vi "PDSS - New Trigger Sequence - Calculate Complete Line Scan.vi"(8 "error in":errorcluster, 9 "FPS":dbl=30.0 format="%0.2p", 10 "Modulation Cycles\nAt Each Wavelength":dbl=1.0 min=1.0 max=30.0 step=1.0, 11 "LCVR Voltages":dbl[][](array[numeric])=[[0.0, 0.0, 0.0, 1.0]]) -> (0 "error out":errorcluster, 1 "LCVR Relaxtion Time":dbl=200.0 format="%#_13g", 3 "AO Graph":waveform(dbl)[](graph)=[{"t0"=timestamp(0 s since 1904-01-01), "dt"=0.000125, "Y"=array[2667 elements]}, {"t0"=timestamp(0 s since 1904-01-01), "dt"=0.000125, "Y"=array[2667 elements]}, {"t0"=timestamp(0 s since 1904-01-01), "dt"=0.000125, "Y"=array[2667 elements]}, {"t0"=timestamp(0 s since 1904-01-01), "dt"=0.000125, "Y"=array[2667 elements]}])   [LabVIEW 2014]
doc: "Build AO waveform for scan."
uses:
  <vilib>/Waveform/WDTOps.llb/WDT Index Channel DBL.vi
  <vilib>/Waveform/WDTOps.llb/WDT Append Waveforms DBL.vi
panel:
  out "Start of First Modulation State - Exposure Relationship 2":waveform(dbl)[](graph)=[{"t0"=timestamp(0 s since 1904-01-01), "dt"=0.000125, "Y"=array[2667 elements]}, {"t0"=timestamp(0 s since 1904-01-01), "dt"=0.000125, "Y"=array[2667 elements]}, {"t0"=timestamp(0 s since 1904-01-01), "dt"=0.000125, "Y"=array[2667 elements]}, {"t0"=timestamp(0 s since 1904-01-01), "dt"=0.000125, "Y"=array[2667 elements]}]
  out "Start of First Modulation State - Exposure Relationship":waveform(dbl)[](graph)=[{"t0"=timestamp(0 s since 1904-01-01), "dt"=0.000125, "Y"=array[2667 elements]}, {"t0"=timestamp(0 s since 1904-01-01), "dt"=0.000125, "Y"=array[2667 elements]}, {"t0"=timestamp(0 s since 1904-01-01), "dt"=0.000125, "Y"=array[2667 elements]}, {"t0"=timestamp(0 s since 1904-01-01), "dt"=0.000125, "Y"=array[2667 elements]}]
  # "There is ALWAYS a 1ms delay at the beginning between the start of a modulation state and the start of a camera exposure.\nThere is ALWAYS a 1.306 ms delay between the end of an exposure and the end of a modulation state."
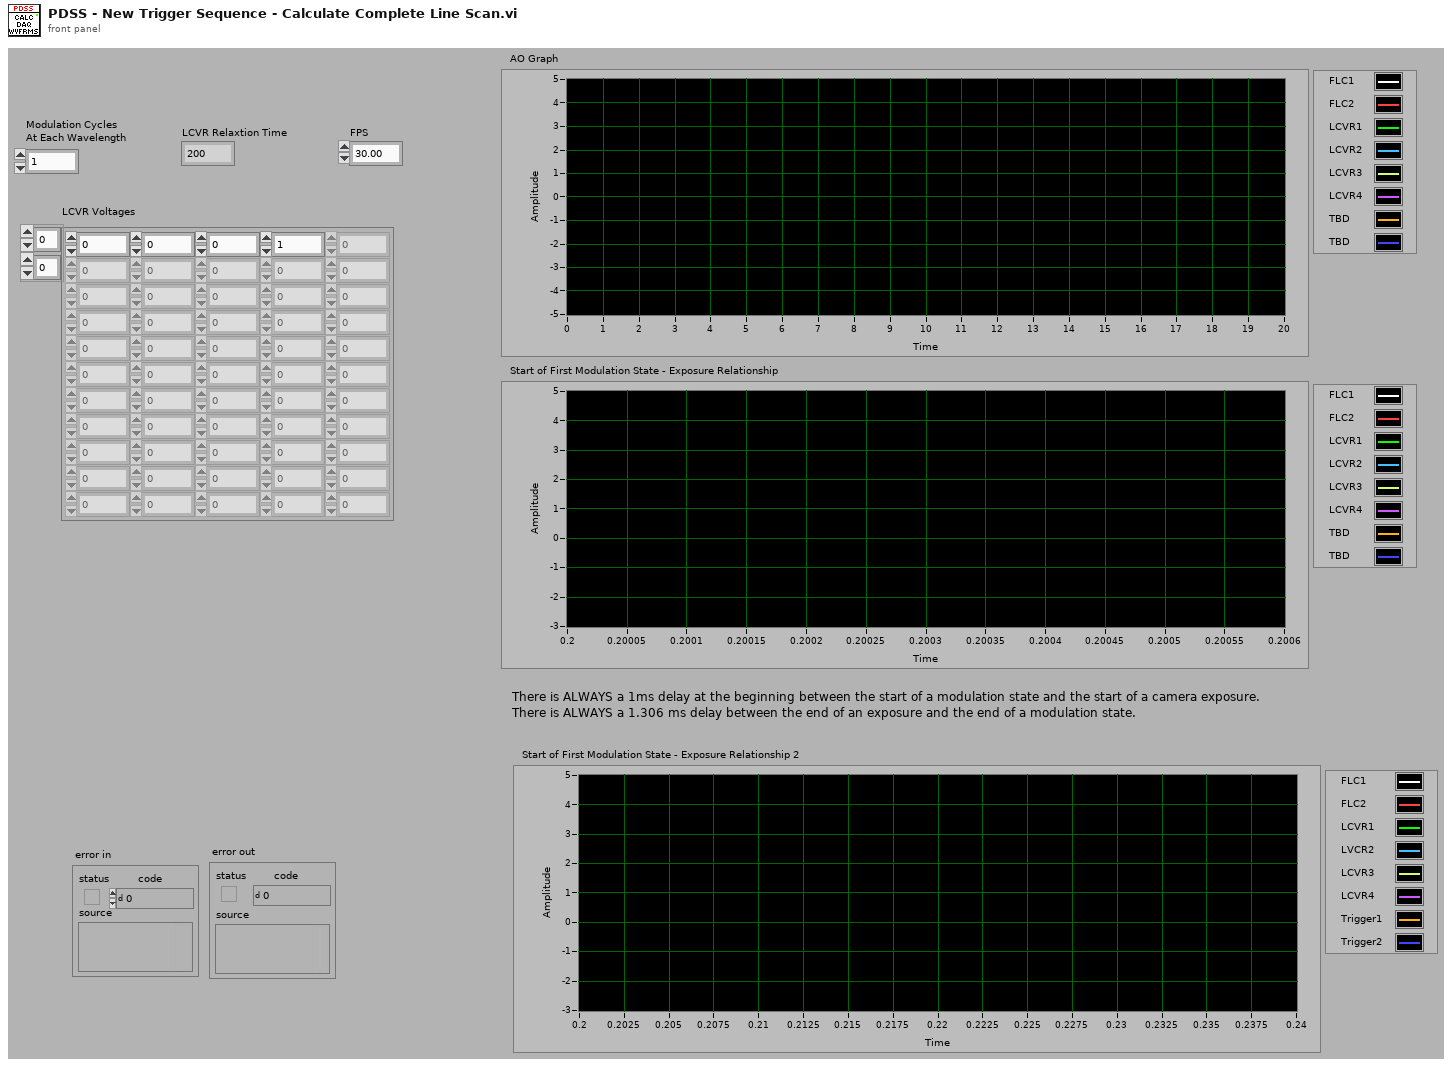
[diagram p1: front panel]
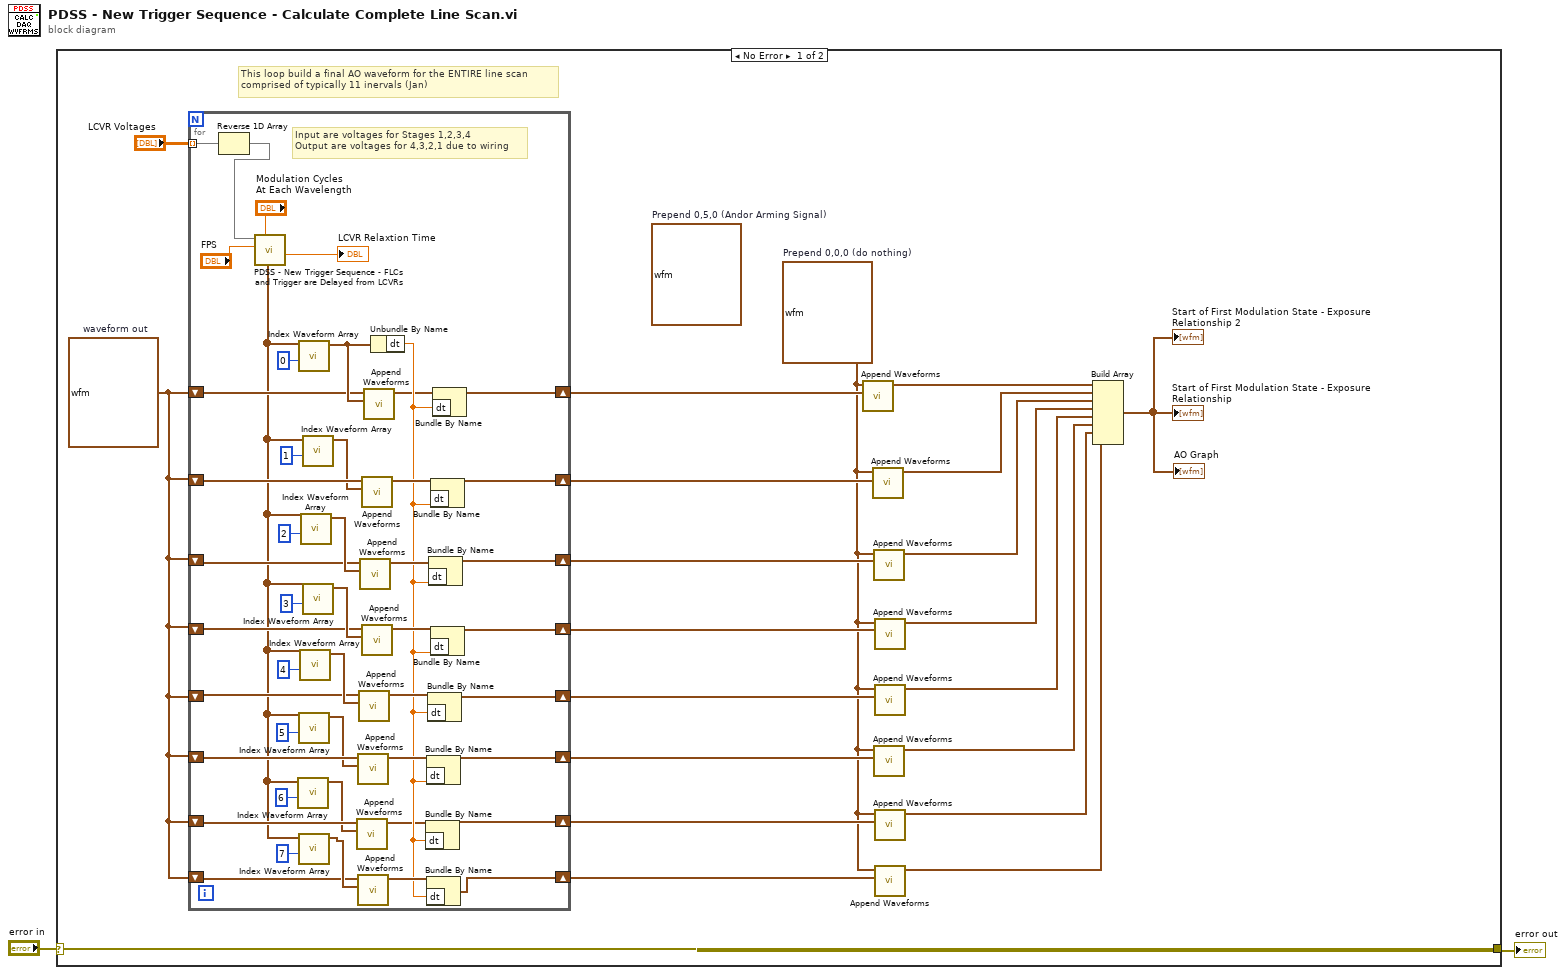
[diagram p0: block diagram]
diagram:
  n1 = case shown="No Error" "error in" {
    selector: "error in" -> [w21 w71]
    tunnel: [w21 w71] -> w1
    frame No Error {
      (unwired) waveform(dbl) {"t0"=timestamp(0 s since 1904-01-01), "dt"=0.000125, "Y"=[0.0, 5.0, 0.0]}  # Prepend 0,5,0 (Andor Arming Signal)
      w3 = waveform(dbl) {"t0"=timestamp(0 s since 1904-01-01), "dt"=0.000125, "Y"=[0.0, 0.0, 0.0]}  # Prepend 0,0,0 (do nothing)
      w23 = waveform(dbl) {"t0"=timestamp(0 s since 1904-01-01), "dt"=1.0, "Y"=[]}  # waveform out
      # "This loop build a final AO waveform for the ENTIRE line scan\ncomprised of typically 11 inervals (Jan)"
      n2 = for {
        shift-right: [w42] -> w12
        shift-left: w23 -> [w31]
        shift-right: [w43] -> w11
        shift-left: w23 -> [w66]
        shift-right: [w44] -> w10
        shift-left: w23 -> [w53]
        shift-right: [w45] -> w9
        shift-left: w23 -> [w52]
        shift-right: [w46] -> w8
        shift-left: w23 -> [w51]
        shift-right: [w47] -> w7
        shift-left: w23 -> [w50]
        tunnel: "LCVR Voltages" -> [w35] mode=indexing
        shift-right: [w48] -> w5
        shift-left: w23 -> [w30]
        shift-right: [w37] -> w6
        shift-left: w23 -> [w38]
        # "Input are voltages for Stages 1,2,3,4\nOutput are voltages for 4,3,2,1 due to wiring"
        n3 = Reverse 1D Array(array=w35) -> (reversed array=w34:dbl[])
        n4 = call "PDSS - New Trigger Sequence - FLCs and Trigger are Delayed from LCVRs.vi"("Modulation Cycles per Wavelength"="Modulation Cycles\nAt Each Wavelength", "FPS"="FPS", "LCVR Tuning Voltages"=w34) -> ("LCVR Relaxtion Time (ms)"=→"LCVR Relaxtion Time":dbl, "AO Waveforms"=w25:waveform(dbl)[])  [unwired: 5 in, 2 out]
        n5 = call-poly <vilib>:"Index Waveform Array.vi"("index"=6, "waveform array"=w25) -> ("waveform"=w28:waveform(dbl))  [unwired: 8 in, 1 out]
        n6 = call-poly <vilib>:"Index Waveform Array.vi"("index"=0, "waveform array"=w25) -> ("waveform"=w69:waveform(dbl))  [unwired: 8 in, 1 out]
        n7 = call-poly <vilib>:"Index Waveform Array.vi"("index"=5, "waveform array"=w25) -> ("waveform"=w27:waveform(dbl))  [unwired: 8 in, 1 out]
        n8 = call-poly <vilib>:"Index Waveform Array.vi"("index"=7, "waveform array"=w25) -> ("waveform"=w40:waveform(dbl))  [unwired: 8 in, 1 out]
        n9 = call-poly <vilib>:"Index Waveform Array.vi"("index"=4, "waveform array"=w25) -> ("waveform"=w54:waveform(dbl))  [unwired: 8 in, 1 out]
        n10 = call-poly <vilib>:"Index Waveform Array.vi"("index"=2, "waveform array"=w25) -> ("waveform"=w56:waveform(dbl))  [unwired: 8 in, 1 out]
        n11 = call-poly <vilib>:"Index Waveform Array.vi"("index"=1, "waveform array"=w25) -> ("waveform"=w65:waveform(dbl))  [unwired: 8 in, 1 out]
        n12 = call-poly <vilib>:"Index Waveform Array.vi"("index"=3, "waveform array"=w25) -> ("waveform"=w55:waveform(dbl))  [unwired: 8 in, 1 out]
        n13 = call-poly <vilib>:"Append Waveforms.vi"("waveform B"=w28, "waveform A"=w30) -> ("waveform out"=w29:waveform(dbl))  [unwired: 8 in, 1 out]
        n14 = call-poly <vilib>:"Append Waveforms.vi"("waveform B"=w27, "waveform A"=w50) -> ("waveform out"=w57:waveform(dbl))  [unwired: 8 in, 1 out]
        n15 = call-poly <vilib>:"Append Waveforms.vi"("waveform B"=w40, "waveform A"=w38) -> ("waveform out"=w41:waveform(dbl))  [unwired: 8 in, 1 out]
        n16 = call-poly <vilib>:"Append Waveforms.vi"("waveform B"=w54, "waveform A"=w51) -> ("waveform out"=w59:waveform(dbl))  [unwired: 8 in, 1 out]
        n17 = call-poly <vilib>:"Append Waveforms.vi"("waveform B"=w56, "waveform A"=w53) -> ("waveform out"=w63:waveform(dbl))  [unwired: 8 in, 1 out]
        n18 = call-poly <vilib>:"Append Waveforms.vi"("waveform B"=w65, "waveform A"=w66) -> ("waveform out"=w67:waveform(dbl))  [unwired: 8 in, 1 out]
        n19 = call-poly <vilib>:"Append Waveforms.vi"("waveform B"=w55, "waveform A"=w52) -> ("waveform out"=w61:waveform(dbl))  [unwired: 8 in, 1 out]
        n20 = call-poly <vilib>:"Append Waveforms.vi"("waveform B"=w69, "waveform A"=w31) -> ("waveform out"=w32:waveform(dbl))  [unwired: 8 in, 1 out]
        n21 = Unbundle By Name(w69) -> ("dt"=w39:dbl)
        n22 = Bundle By Name(cluster=w29, "dt"=w39) -> (w48:waveform(dbl))
        n23 = Bundle By Name(cluster=w57, "dt"=w39) -> (w47:waveform(dbl))
        n24 = Bundle By Name(cluster=w41, "dt"=w39) -> (w37:waveform(dbl))
        n25 = Bundle By Name(cluster=w59, "dt"=w39) -> (w46:waveform(dbl))
        n26 = Bundle By Name(cluster=w63, "dt"=w39) -> (w44:waveform(dbl))
        n27 = Bundle By Name(cluster=w67, "dt"=w39) -> (w43:waveform(dbl))
        n28 = Bundle By Name(cluster=w61, "dt"=w39) -> (w45:waveform(dbl))
        n29 = Bundle By Name(cluster=w32, "dt"=w39) -> (w42:waveform(dbl))
      }
      n30 = call-poly <vilib>:"Append Waveforms.vi"("waveform B"=w12, "waveform A"=w3) -> ("waveform out"=w13:waveform(dbl))  [unwired: 8 in, 1 out]
      n31 = call-poly <vilib>:"Append Waveforms.vi"("waveform B"=w11, "waveform A"=w3) -> ("waveform out"=w20:waveform(dbl))  [unwired: 8 in, 1 out]
      n32 = call-poly <vilib>:"Append Waveforms.vi"("waveform B"=w10, "waveform A"=w3) -> ("waveform out"=w19:waveform(dbl))  [unwired: 8 in, 1 out]
      n33 = call-poly <vilib>:"Append Waveforms.vi"("waveform B"=w7, "waveform A"=w3) -> ("waveform out"=w17:waveform(dbl))  [unwired: 8 in, 1 out]
      n34 = call-poly <vilib>:"Append Waveforms.vi"("waveform B"=w9, "waveform A"=w3) -> ("waveform out"=w18:waveform(dbl))  [unwired: 8 in, 1 out]
      n35 = call-poly <vilib>:"Append Waveforms.vi"("waveform B"=w8, "waveform A"=w3) -> ("waveform out"=w16:waveform(dbl))  [unwired: 8 in, 1 out]
      n36 = call-poly <vilib>:"Append Waveforms.vi"("waveform B"=w5, "waveform A"=w3) -> ("waveform out"=w15:waveform(dbl))  [unwired: 8 in, 1 out]
      n37 = call-poly <vilib>:"Append Waveforms.vi"("waveform B"=w6, "waveform A"=w3) -> ("waveform out"=w14:waveform(dbl))  [unwired: 8 in, 1 out]
      n38 = Build Array(w13, w20, w19, w18, w16, w17, w15, w14) -> (→"AO Graph" →"Start of First Modulation State - Exposure Relationship" →"Start of First Modulation State - Exposure Relationship 2":waveform(dbl)[])
    }
    frame Error {
    }
  }
  "error out" <- w1
